vi "InitShell.vi"(10 "error out 2":errorcluster) -> (3 "error out":errorcluster, 4 "String":string)   [LabVIEW 2011]
uses:
  Variables/CameraStatus.vi
  Variables/ScannerMirrorStatus.vi
  Variables/AOTFStatus.vi
  Variables/KoherasStatus.vi
  Variables/GlobalGetCamerasOnOff.vi
  Variables/GlobalGetPhysikalInstrumentsOnOff.vi
  Variables/GlobalGetAOTFOnOff.vi
  Variables/GlobalGetKoherasLaserOnOff.vi
  Variables/GlobalGetTemperatureCamera.vi
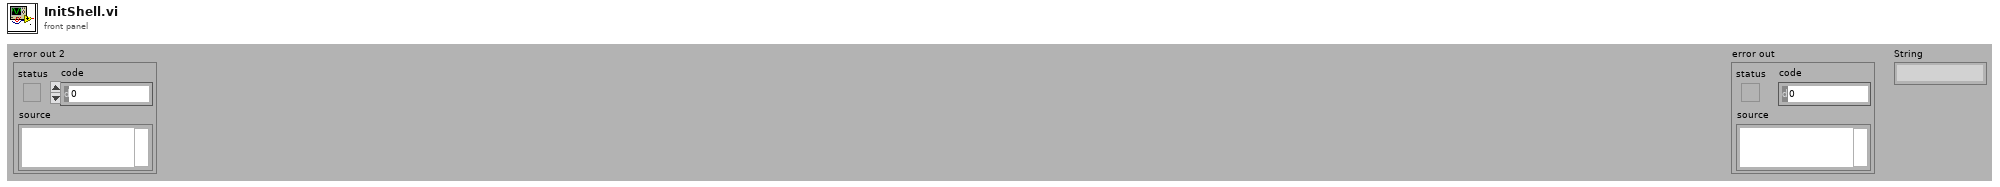
[diagram p1: front panel]
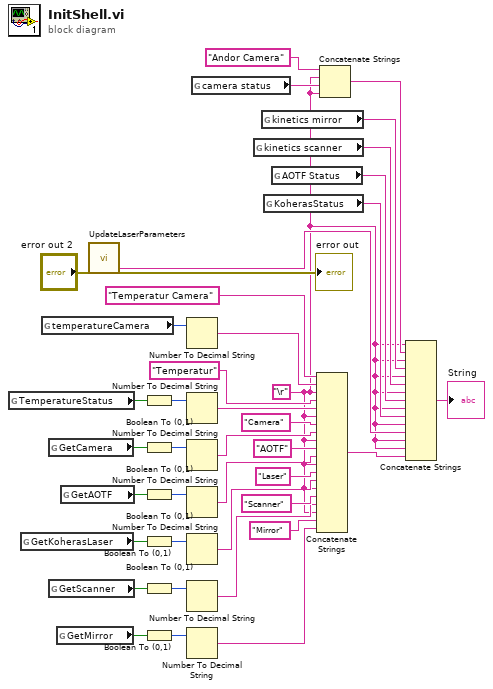
[diagram p0: block diagram]
diagram:
  w1 = "\r"
  n1 = global read "GlobalGetTemperatureCamera.vi" "TemperatureStatus"() -> (w28:bool)
  n2 = global read "GlobalGetKoherasLaserOnOff.vi" "GetKoherasLaser"() -> (w14:bool)
  n3 = global read "GlobalGetTemperatureCamera.vi" "temperatureCamera"() -> (w30:i32)
  n4 = global read "GlobalGetCamerasOnOff.vi" "GetCamera"() -> (w24:bool)
  n5 = global read "GlobalGetPhysikalInstrumentsOnOff.vi" "GetScanner"() -> (w10:bool)
  n6 = global read "GlobalGetPhysikalInstrumentsOnOff.vi" "GetMirror"() -> (w6:bool)
  n7 = global read "GlobalGetAOTFOnOff.vi" "GetAOTF"() -> (w18:bool)
  n8 = call "UpdateLaserParameters.vi"("error in"="error out 2") -> ("ToShell"=w39:string, "error out"=→"error out":errorcluster)  [unwired: 23 in, 2 out]
  n9 = Boolean To (0,1)(Boolean=w28) -> (0, 1=w27:i16)
  n10 = Boolean To (0,1)(Boolean=w24) -> (0, 1=w22:i16)
  n11 = Boolean To (0,1)(Boolean=w18) -> (0, 1=w19:i16)
  n12 = Boolean To (0,1)(Boolean=w14) -> (0, 1=w15:i16)
  n13 = Boolean To (0,1)(Boolean=w10) -> (0, 1=w13:i16)
  n14 = Boolean To (0,1)(Boolean=w6) -> (0, 1=w8:i16)
  n15 = Number To Decimal String(number=w30) -> (decimal integer string=w31:string)  [unwired: 1 in]
  n16 = Number To Decimal String(number=w27) -> (decimal integer string=w26:string)  [unwired: 1 in]
  n17 = Number To Decimal String(number=w22) -> (decimal integer string=w23:string)  [unwired: 1 in]
  n18 = Number To Decimal String(number=w19) -> (decimal integer string=w20:string)  [unwired: 1 in]
  n19 = Number To Decimal String(number=w15) -> (decimal integer string=w16:string)  [unwired: 1 in]
  n20 = Number To Decimal String(number=w13) -> (decimal integer string=w11:string)  [unwired: 1 in]
  n21 = Number To Decimal String(number=w8) -> (decimal integer string=w7:string)  [unwired: 1 in]
  n22 = global read "CameraStatus.vi" "camera status"() -> (w2:string)
  n23 = global read "ScannerMirrorStatus.vi" "kinetics scanner"() -> (w33:string)
  n24 = global read "ScannerMirrorStatus.vi" "kinetics mirror"() -> (w34:string)
  n25 = global read "KoherasStatus.vi" "KoherasStatus"() -> (w36:string)
  n26 = global read "AOTFStatus.vi" "AOTF Status"() -> (w37:string)
  n27 = Concatenate Strings("Temperatur Camera" ("string"), w31, w1, "Temperatur" ("string"), w26, w1, "Camera" ("string"), w23, w1, "AOTF" ("string"), w20, w1, "Laser" ("string"), w16, w1, "Scanner" ("string"), w11, w1, "Mirror" ("string"), w7) -> (w5:string)
  n28 = Concatenate Strings("Andor Camera" ("string"), w1, w2, w1) -> (w40:string)
  n29 = Concatenate Strings(w1, w40, w1, w34, w1, w33, w1, w37, w1, w36, w1, w39, w1, w1, w5) -> (→"String":string)
